vi "MULTTCP_AsyncHandler.vi"(0 "async_on_block":refnum<vi>, 1 "last async ref":refnum<vi>, 5 "block notifier":refnum<notifier>, 7 "asyncN":refnum<notifier>, 9 "async notifier":refnum<notifier>, 11 "error async out":errorcluster, 12 "async reference":refnum<vi>, 13 "logfile":path, 14 "Log":bool=TRUE) -> (15 "error async out":errorcluster)   [LabVIEW 2016]
uses:
  DBSHAND/private/vis/DatabaseHand_Element_Get(string).vi
panel:
  out "error out":errorcluster
  in  "async_on_block 2":bool
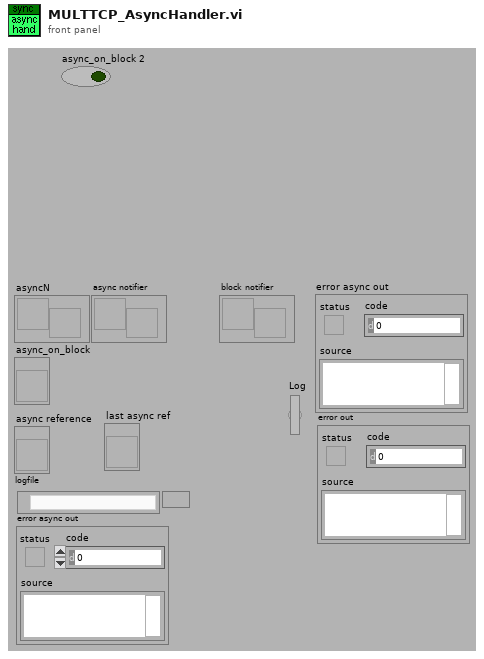
[diagram p1: front panel]
types:
  T1 = typedef "DatabaseHand_RefNum.ctl" = refnum<vi>
  T2 = typedef "MULTTCP_BlockingStruct.ctl" = cluster{"cmd":string, "message back  queue":refnum<queue>}
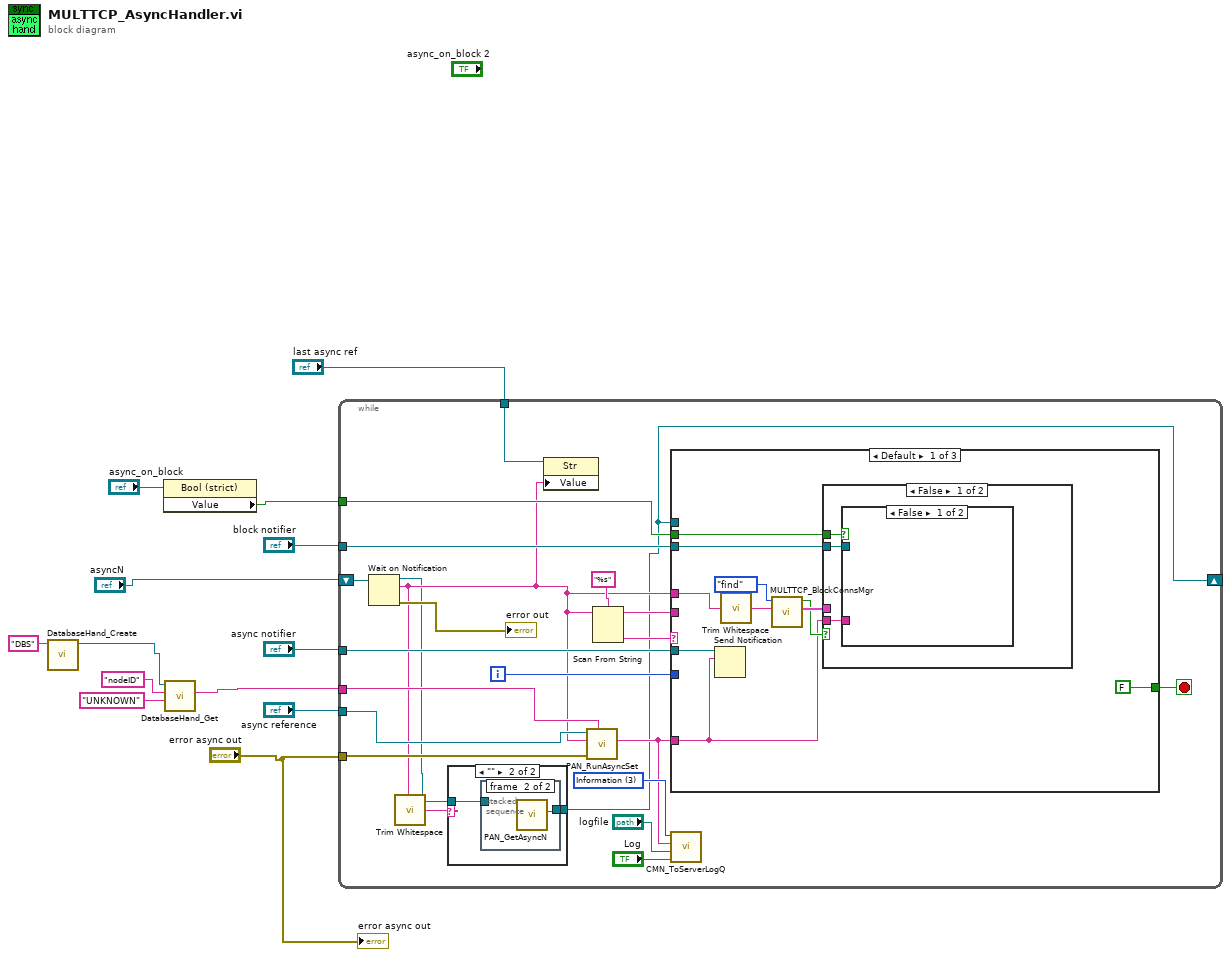
[diagram p0: block diagram]
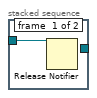
[diagram p3: hidden frame]
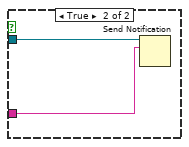
[diagram p4: hidden frame]
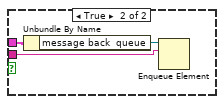
[diagram p5: hidden frame]
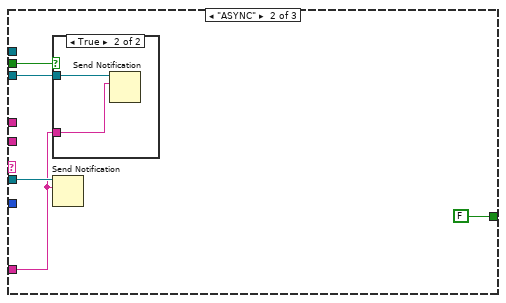
[diagram p6: hidden frame]
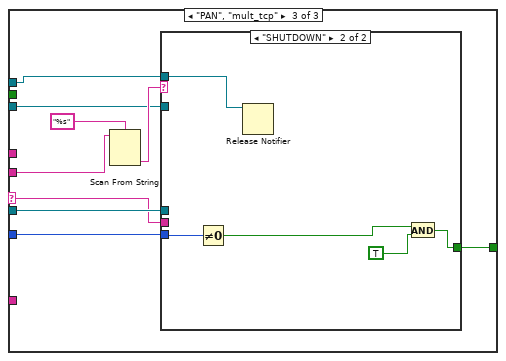
[diagram p8: hidden frame]
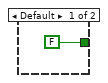
[diagram p9: hidden frame]
diagram:
  n1 = call "DatabaseHand_Create.vi"("Name"="DBS") -> ("Database RefNum out"=w3:T1)  [unwired: 1 in, 9 out]
  n2 = property class="Bool (strict)"(reference="async_on_block") -> ("Value"=w6:bool)  [unwired: 1 in, 2 out]
  n3 = call-poly "DatabaseHand_Get.vi"("default value"="UNKNOWN", "name"="nodeID", "Database RefNum in"=w3) -> ("value"=w2:string)  [unwired: 2 in, 6 out]
  n4 = while {
    tunnel: "async notifier" -> [w32]
    tunnel: "block notifier" -> [w29]
    tunnel: "async reference" -> [w28]
    tunnel: "error async out" -> [w27]
    tunnel: w6 -> [w25]
    tunnel: "last async ref" -> [w22]
    tunnel: w2 -> [w21]
    shift-right: [w14] -> _
    shift-left: "asyncN" -> [w15]
    i -> [w20]
    stop <- w33 stop-if-true
    w30 = u16 3 items=["command", "imediateReply", "Callback Reply", "Information", "none"] ("type")
    n5 = Wait on Notification(notifier=w15) -> (notifier out=w16:refnum<notifier>, notification=w18:string, error out=→"error out":errorcluster)  [unwired: 1 in, 3 out]
    n6 = call <vilib>:"Trim Whitespace.vi"("string"=w18) -> ("trimmed string"=w17:string)  [unwired: 1 in]
    n7 = case shown="\"\"" w17 {
      tunnel: w16 -> [w36 w38]
      tunnel: [w36 w37] -> w14
      frame Default {
      }
      frame "" {
        n8 = stacked-sequence {
          tunnel: w38 -> [w39 _]
          tunnel: [_ w40] -> w37
          frame #0 {
            n9 = Release Notifier(notifier=w39) -> ()  [unwired: 1 in, 4 out]
          }
          frame #1 {
            n10 = call "PAN_GetAsyncN.vi"() -> ("asyncN"=w40:refnum<notifier>)  [unwired: 11 out]
          }
        }
      }
    }
    n11 = property class="Str"(reference=w22, "Value"=w18) -> ()  [unwired: 1 in, 2 out]
    n12 = call "PAN_RunAsyncSet.vi"("nodeID"=w21, "error in (no error)"=w27, "msg in"=w18, "type specifier VI Refnum (for type only)"=w28) -> ("resp out"=w26:string)  [unwired: 7 out]
    n13 = Scan From String(format string="%s", input string=w18) -> (remaining string=w31:string, output 1=w34:string)  [unwired: 2 in, 3 out]
    n14 = case shown="Default" w34 {
      selector: w34 -> [_ _ w73]
      tunnel: [FALSE FALSE w69] -> w33
      tunnel: w32 -> [w43 w62 w74]
      tunnel: w18 -> [w47 _ _]
      tunnel: w14 -> [_ _ w67]
      tunnel: w31 -> [_ _ w72]
      tunnel: w29 -> [w42 w61 w68]
      tunnel: w26 -> [w44 w60 _]
      tunnel: w25 -> [w41 w59 _]
      tunnel: w20 -> [_ _ w66]
      frame Default {
        n15 = Send Notification(notification=w44, notifier=w43) -> ()  [unwired: 1 in, 2 out]
        n16 = call <vilib>:"Trim Whitespace.vi"("string"=w47) -> ("trimmed string"=w46:string)  [unwired: 1 in]
        n17 = call "MULTTCP_BlockConnsMgr.vi"("arg"=w46, "action"=enum16{"add", "delete", "find"}."find") -> ("connection out"=w49:T2, "send CB"=w45:bool)  [unwired: 2 in, 6 out]
        n18 = case shown="False" w45 {
          tunnel: w49 -> [_ w58]
          tunnel: w44 -> [w52 w56]
          tunnel: w42 -> [w53 _]
          tunnel: w41 -> [w51 _]
          frame False {
            n19 = case shown="False" w51 {
              tunnel: w53 -> [_ w55]
              tunnel: w52 -> [_ w54]
              frame False {
              }
              frame True {
                n20 = Send Notification(notification=w54, notifier=w55) -> ()  [unwired: 1 in, 2 out]
              }
            }
          }
          frame True {
            n21 = Unbundle By Name(w58) -> ("message back  queue"=w57:refnum<queue>)
            n22 = Enqueue Element(queue=w57, element=w56) -> ()  [unwired: 1 in, 4 out]
          }
        }
      }
      frame "ASYNC" {
        n23 = case shown="True" w59 {
          tunnel: w61 -> [_ w65]
          tunnel: w60 -> [_ w64]
          frame False {
          }
          frame True {
            n24 = Send Notification(notification=w64, notifier=w65) -> ()  [unwired: 1 in, 2 out]
          }
        }
        n25 = Send Notification(notification=w60, notifier=w62) -> ()  [unwired: 1 in, 2 out]
      }
      frame "PAN", "mult_tcp" {
        n26 = Scan From String(format string="%s", input string=w72) -> (output 1=w70:string)  [unwired: 2 in, 4 out]
        n27 = case shown="\"SHUTDOWN\"" w70 {
          tunnel: w74 -> [_ _]
          tunnel: w73 -> [_ _]
          tunnel: [FALSE w78] -> w69
          tunnel: w68 -> [_ _]
          tunnel: w67 -> [_ w80]
          tunnel: w66 -> [_ w77]
          frame Default {
          }
          frame "SHUTDOWN" {
            n28 = Not Equal To 0?(x=w77) -> (x != 0?=w76:bool)
            n29 = Release Notifier(notifier=w80) -> ()  [unwired: 1 in, 4 out]
            n30 = And(x=w76, y=TRUE) -> (x .and. y?=w78:bool)
          }
        }
      }
    }
    n31 = call "CMN_ToServerLogQ.vi"("Log"="Log", "file"="logfile", "string"=w26, "type"=w30) -> ()  [unwired: 2 in, 5 out]
  }
  "error async out" <- "error async out"
